vi "子界面-评定报告生成.vi"(0 "产品序号":string, 1 "测试人":string, 2 "部位":string, 3 "总面积":i32) -> (7 "写入数据库路径":path)   [LabVIEW 2018]
uses:
  <vilib>/Utility/NIReport.llb/Report Type.ctl
  <vilib>/addons/database/Connection.llb/DB Tools Open Connec (String).vi
  <vilib>/Utility/NIReport.llb/Append Report Text (str wrap).vi
  <vilib>/Utility/NIReport.llb/Append Report Text (num wrap).vi
  <vilib>/addons/database/_DB Variant To Data/Database Variant To Data.xnode
  <vilib>/Utility/NIReport.llb/NI_report.lvclass
  <vilib>/addons/database/NI_Database_API.lvlib
  <vilib>/Utility/NIReport.llb/NI_ReportGenerationCore.lvlib
panel:
  out "报告生成路径":path
  out "最大Z值":cluster{dbl}
  out "评定等级":string
  out "data":T1
  out "评定等级2":string caption="评定等级"
  out "缺陷占比(%)":dbl
  out "数值":dbl
  in  "返回 2":bool
  out "data 2":T1
  # "评定和分级结果"
  # "分层类"
  # "弥散类"
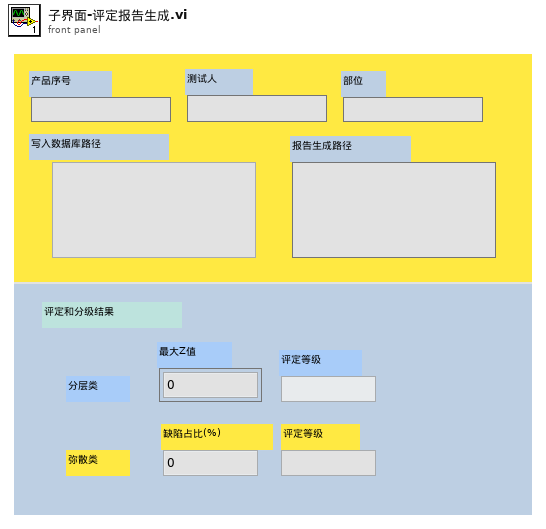
[diagram p1: front panel]
types:
  T1 = typedef "Z值ctl.ctl" = cluster{dbl}[]
  T2 = cluster{"position (Excel)":cluster{"row":i32, "column":i32}, "name (Excel)":string, "bookmark (Word)":string}
  T3 = typedef "NI_ReportGenerationCore.lvlib/Report Type.ctl" = enum16{"HTML", "Word", "Excel"}
  T4 = typedef "NI_Database_API.lvlib/Conn ObjectReference.ctl" = refnum<k1>
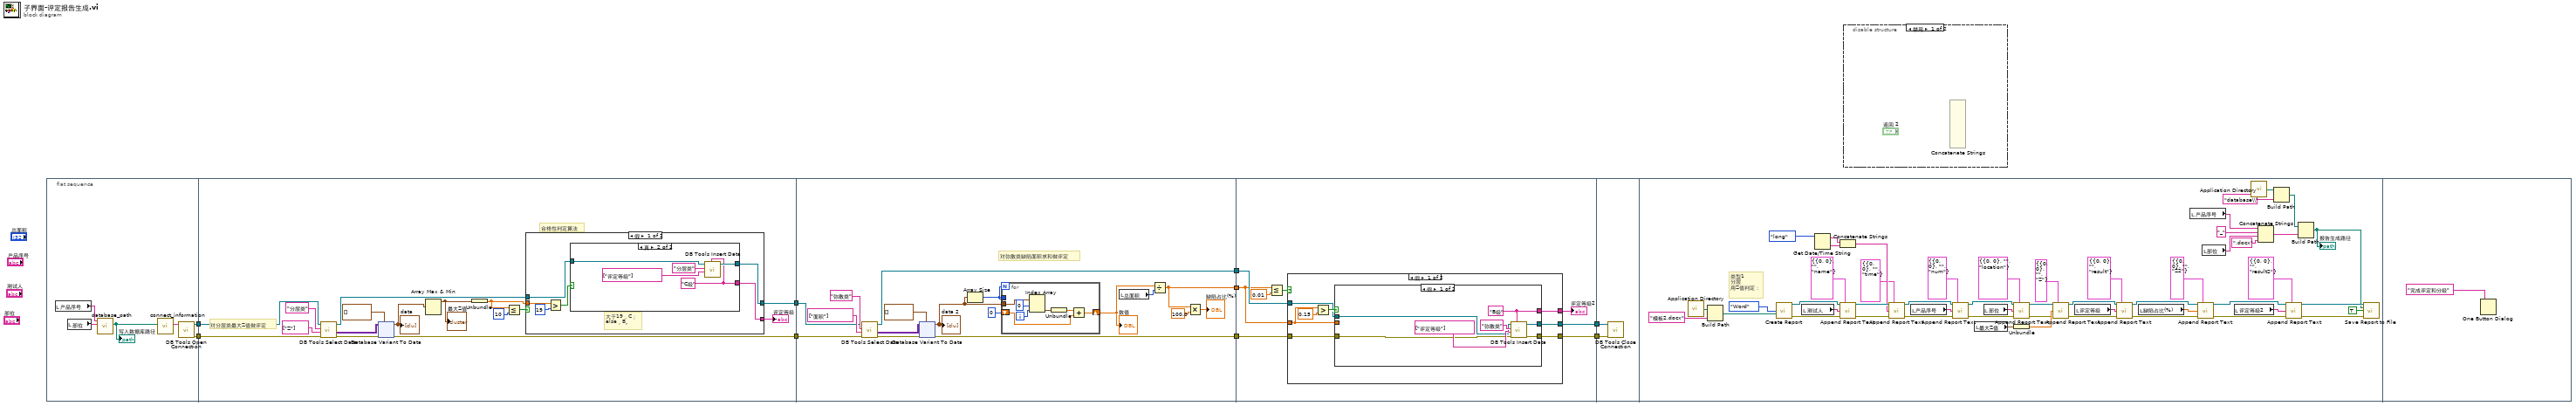
[diagram p0: block diagram]
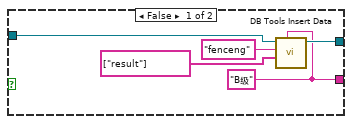
[diagram p2: hidden frame]
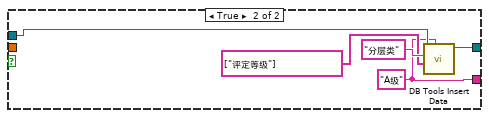
[diagram p3: hidden frame]
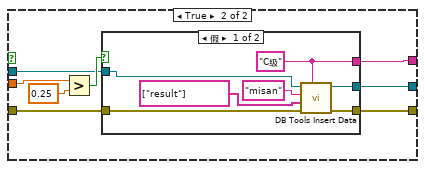
[diagram p4: hidden frame]
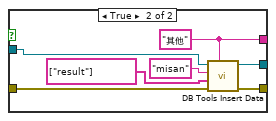
[diagram p5: hidden frame]
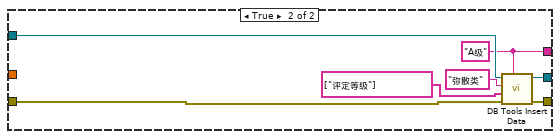
[diagram p6: hidden frame]
diagram:
  n1 = flat-sequence {
    tunnel: [w11] -> w9
    tunnel: [w10] -> w8
    tunnel: w9 -> [w25]
    tunnel: w8 -> [w28]
    tunnel: [w19] -> w7
    tunnel: [w17] -> w6
    tunnel: [w104] -> w5
    tunnel: w7 -> [w108]
    tunnel: w6 -> [w105]
    tunnel: [w103] -> w4
    tunnel: [w96] -> w3
    tunnel: w5 -> [w162]
    tunnel: w4 -> [w164]
    tunnel: [w163] -> w2
    tunnel: [w161] -> w1
    tunnel: w3 -> [w160]
    tunnel: w2 -> [w212]
    tunnel: w1 -> [w211]
    frame #0 {
      n2 = local read "产品序号"() -> (w13:string)
      n3 = local read "部位"() -> (w12:string)
      n4 = call "database_path.vi"("部位"=w12, "产品序号"=w13) -> ("database path"=w14:path)  [unwired: 9 in]
      "写入数据库路径" <- w14
      n5 = call "connect_information.vi"("路径"=w14) -> ("connect info"=w15:string)  [unwired: 10 in]
      n6 = call-poly <vilib>:"DB Tools Open Connection.vi"("connection information"=w15) -> ("error out"=w10:errorcluster, "connection reference"=w11:T4)  [unwired: 7 in]
    }
    frame #1 {
      # "合格性判定算法"
      # "对分层类最大Z值做评定"
      n7 = call <vilib>:"DB Tools Select Data.vi"("error in (no error)"=w28, "columns"=string[] ["Z"], "table"="分层类", "connection reference"=w25) -> ("error out"=w29:errorcluster, "data"=w27:variant[][], "connection reference out"=w20:T4)  [unwired: 2 in]
      n8 = xnode "Database Variant To Data"("database variant"=w27, "error in (no error)"=w29, "type"=T1 []) -> ("data"=w24:T1, "error out"=w17:errorcluster)
      "data" <- w24
      n9 = Array Max & Min(array=w24) -> (max value=w21:cluster{dbl})  [unwired: 3 out]
      "最大Z值" <- w21
      n10 = Unbundle(w21) -> (w18:dbl)
      n11 = Less Or Equal?(x=w18, y=10) -> (x <= y?=w22:bool)
      n12 = case shown="假" w22 {
        tunnel: w20 -> [w35 w52]
        tunnel: [w34 w49] -> w19
        tunnel: w18 -> [w33 _]
        tunnel: [w32 w48] -> w16
        frame False {
          # "大于19，C；\nelse，B。"
          n13 = Greater?(x=w33, y=19) -> (0:w36:bool)
          n14 = case shown="真" w36 {
            tunnel: w35 -> [w40 w44]
            tunnel: [w39 w45] -> w34
            tunnel: [w38 w43] -> w32
            frame False {
              w38 = "B级"
              n15 = call <vilib>:"DB Tools Insert Data.vi"("data"=w38, "columns"=string[] ["result"], "table"="fenceng", "connection reference"=w40) -> ("connection reference out"=w39:T4)  [unwired: 6 in, 1 out]
            }
            frame True {
              w43 = "C级"
              n16 = call <vilib>:"DB Tools Insert Data.vi"("data"=w43, "columns"=string[] ["评定等级"], "table"="分层类", "connection reference"=w44) -> ("connection reference out"=w45:T4)  [unwired: 6 in, 1 out]
            }
          }
        }
        frame True {
          w48 = "A级"
          n17 = call <vilib>:"DB Tools Insert Data.vi"("data"=w48, "columns"=string[] ["评定等级"], "table"="分层类", "connection reference"=w52) -> ("connection reference out"=w49:T4)  [unwired: 6 in, 1 out]
        }
      }
      "评定等级" <- w16
    }
    frame #2 {
      # "对弥散类缺陷面积求和做评定"
      n18 = call <vilib>:"DB Tools Select Data.vi"("error in (no error)"=w105, "columns"=string[] ["面积"], "table"="弥散类", "connection reference"=w108) -> ("error out"=w106:errorcluster, "data"=w107:variant[][], "connection reference out"=w103:T4)  [unwired: 2 in]
      n19 = xnode "Database Variant To Data"("database variant"=w107, "error in (no error)"=w106, "type"=T1 []) -> ("data"=w101:T1, "error out"=w104:errorcluster)
      "data 2" <- w101
      n20 = Array Size(array=w101) -> (size(s)=w100:i32)
      n21 = for {
        N: w100 -> [_]
        tunnel: w101 -> [w117]
        tunnel: w100 -> [_]
        shift-right: [w112] -> w98
        shift-left: 0 -> [w111]
        i -> [w115]
        n22 = Index Array(array=w117, index #1=0 ("索引 (列)"), index #2=w115) -> (element #2=w114:cluster{dbl})  [unwired: 1 out]
        n23 = Unbundle(w114) -> (w113:dbl)
        n24 = Add(x=w113, y=w111) -> (x+y=w112:dbl)
      }
      "数值" <- w98
      n25 = local read "总面积"() -> (w97:i32)
      n26 = Divide(x=w98, y=w97) -> (x/y=w96:dbl)
      n27 = Multiply(x=w96, y=100.0) -> (x*y=→"缺陷占比(%)":dbl)
    }
    frame #3 {
      n28 = Less Or Equal?(x=w160, y=0.01) -> (x <= y?=w166:bool)
      n29 = case shown="假" w166 {
        tunnel: w164 -> [w171 w208]
        tunnel: [w170 w207] -> w163
        tunnel: w162 -> [w168 w206]
        tunnel: [w169 w205] -> w161
        tunnel: w160 -> [w172 _]
        tunnel: [w167 w204] -> w159
        frame False {
          n30 = Greater?(x=w172, y=0.15) -> (0:w173:bool)
          n31 = case shown="假" w173 {
            tunnel: w172 -> [_ w187]
            tunnel: w171 -> [w179 w186]
            tunnel: [w178 w185] -> w170
            tunnel: [w177 w184] -> w169
            tunnel: w168 -> [w176 w183]
            tunnel: [w175 w182] -> w167
            frame False {
              w175 = "B级"
              n32 = call <vilib>:"DB Tools Insert Data.vi"("data"=w175, "error in (no error)"=w176, "columns"=string[] ["评定等级"], "table"="弥散类", "connection reference"=w179) -> ("error out"=w177:errorcluster, "connection reference out"=w178:T4)  [unwired: 5 in]
            }
            frame True {
              n33 = Greater?(x=w187, y=0.25) -> (0:w188:bool)
              n34 = case shown="假" w188 {
                tunnel: w186 -> [w194 w201]
                tunnel: [w193 w200] -> w185
                tunnel: [w192 w199] -> w184
                tunnel: w183 -> [w191 w198]
                tunnel: [w190 w197] -> w182
                frame False {
                  w190 = "C级"
                  n35 = call <vilib>:"DB Tools Insert Data.vi"("data"=w190, "error in (no error)"=w191, "columns"=string[] ["result"], "table"="misan", "connection reference"=w194) -> ("error out"=w192:errorcluster, "connection reference out"=w193:T4)  [unwired: 5 in]
                }
                frame True {
                  w197 = "其他"
                  n36 = call <vilib>:"DB Tools Insert Data.vi"("data"=w197, "error in (no error)"=w198, "columns"=string[] ["result"], "table"="misan", "connection reference"=w201) -> ("error out"=w199:errorcluster, "connection reference out"=w200:T4)  [unwired: 5 in]
                }
              }
            }
          }
        }
        frame True {
          w204 = "A级"
          n37 = call <vilib>:"DB Tools Insert Data.vi"("data"=w204, "error in (no error)"=w206, "columns"=string[] ["评定等级"], "table"="弥散类", "connection reference"=w208) -> ("error out"=w205:errorcluster, "connection reference out"=w207:T4)  [unwired: 5 in]
        }
      }
      "评定等级2" <- w159
    }
    frame #4 {
      n38 = call <vilib>:"DB Tools Close Connection.vi"("error in (no error)"=w211, "connection reference"=w212) -> ()  [unwired: 5 in, 1 out]
    }
    frame #5 {
      # "类型1\n分层\n用Z值判定："
      n39 = call <vilib>:"Application Directory.vi"() -> ("Application Directory"=w264:path)
      n40 = Build Path(base path=w264, name or relative path="模板2.docx") -> (appended path=w263:path)
      n41 = call <vilib>:"Create Report.vi"("report type"=Report_Type."Word" ("Report Type"), "template (empty)"=w263) -> ("report out"=w246:refnum<class "NI_report.lvclass">, "error out"=w245:errorcluster)  [unwired: 12 in]
      n42 = local read "测试人"() -> (w244:string)
      n43 = Get Date/Time String(date format (0)=enum16{"short", "long", "abbreviated"}."long" ("日期格式(0)")) -> (date string=w252:string, time string=w254:string)  [unwired: 2 in]
      n44 = Concatenate Strings(w252, w254) -> (w253:string)
      n45 = call-poly <vilib>:"Append Report Text.vi"("report in"=w246, "MS Office parameters"=T2 {"position (Excel)"={"row"=0, "column"=0}, "name (Excel)"="", "bookmark (Word)"="name"}, "text"=w244, "error in (no error)"=w245) -> ("report out"=w257:refnum<class "NI_report.lvclass">, "error out"=w258:errorcluster)  [unwired: 8 in, 2 out]
      n46 = call-poly <vilib>:"Append Report Text.vi"("report in"=w257, "MS Office parameters"=T2 {"position (Excel)"={"row"=0, "column"=0}, "name (Excel)"="", "bookmark (Word)"="time"}, "text"=w253, "error in (no error)"=w258) -> ("report out"=w255:refnum<class "NI_report.lvclass">, "error out"=w256:errorcluster)  [unwired: 8 in, 2 out]
      n47 = local read "产品序号"() -> (w243:string)
      n48 = call-poly <vilib>:"Append Report Text.vi"("report in"=w255, "MS Office parameters"=T2 {"position (Excel)"={"row"=0, "column"=0}, "name (Excel)"="", "bookmark (Word)"="num"}, "text"=w243, "error in (no error)"=w256) -> ("report out"=w259:refnum<class "NI_report.lvclass">, "error out"=w260:errorcluster)  [unwired: 8 in, 2 out]
      n49 = local read "最大Z值"() -> (w236:cluster{dbl})
      n50 = local read "部位"() -> (w242:string)
      n51 = call-poly <vilib>:"Append Report Text.vi"("report in"=w259, "MS Office parameters"=T2 {"position (Excel)"={"row"=0, "column"=0}, "name (Excel)"="", "bookmark (Word)"="location"}, "text"=w242, "error in (no error)"=w260) -> ("report out"=w232:refnum<class "NI_report.lvclass">, "error out"=w231:errorcluster)  [unwired: 8 in, 2 out]
      n52 = Unbundle(w236) -> (w237:dbl)
      n53 = call-poly <vilib>:"Append Report Text.vi"("report in"=w232, "MS Office parameters"=T2 {"position (Excel)"={"row"=0, "column"=0}, "name (Excel)"="", "bookmark (Word)"="Z"}, "text"=w237, "error in (no error)"=w231) -> ("report out"=w230:refnum<class "NI_report.lvclass">, "error out"=w229:errorcluster)  [unwired: 8 in, 2 out]
      n54 = local read "评定等级"() -> (w235:string)
      n55 = call-poly <vilib>:"Append Report Text.vi"("report in"=w230, "MS Office parameters"=T2 {"position (Excel)"={"row"=0, "column"=0}, "name (Excel)"="", "bookmark (Word)"="result"}, "text"=w235, "error in (no error)"=w229) -> ("report out"=w228:refnum<class "NI_report.lvclass">, "error out"=w227:errorcluster)  [unwired: 8 in, 2 out]
      n56 = local read "缺陷占比(%)"() -> (w234:dbl)
      n57 = local read "产品序号"() -> (w220:string)
      n58 = call-poly <vilib>:"Append Report Text.vi"("report in"=w228, "MS Office parameters"=T2 {"position (Excel)"={"row"=0, "column"=0}, "name (Excel)"="", "bookmark (Word)"="Z2"}, "text"=w234, "error in (no error)"=w227) -> ("report out"=w226:refnum<class "NI_report.lvclass">, "error out"=w225:errorcluster)  [unwired: 8 in, 2 out]
      n59 = local read "部位"() -> (w219:string)
      n60 = local read "评定等级2"() -> (w233:string)
      n61 = call <vilib>:"Application Directory.vi"() -> ("Application Directory"=w215:path)
      n62 = Concatenate Strings(w220, "_" ("名称或相对路径"), w219, ".docx" ("名称或相对路径")) -> (w223:string)
      n63 = Build Path(base path=w215, name or relative path="database\\" ("名称或相对路径")) -> (appended path=w213:path)
      n64 = call-poly <vilib>:"Append Report Text.vi"("report in"=w226, "MS Office parameters"=T2 {"position (Excel)"={"row"=0, "column"=0}, "name (Excel)"="", "bookmark (Word)"="result2"}, "text"=w233, "error in (no error)"=w225) -> ("report out"=w218:refnum<class "NI_report.lvclass">, "error out"=w217:errorcluster)  [unwired: 8 in, 2 out]
      n65 = Build Path(base path=w213, name or relative path=w223) -> (appended path=w216:path)
      "报告生成路径" <- w216
      n66 = call-dynamic "Save Report to File.vi"("report in"=w218, "report file path"=w216, "prompt to replace? (F)"=TRUE, "error in (no error)"=w217) -> ()  [unwired: 10 in, 2 out]
    }
    frame #6 {
      n67 = One Button Dialog(message="完成评定和分级" ("消息")) -> ()  [unwired: 1 in, 1 out]
    }
  }
  n68 = disable-structure shown="禁用" {
    frame Disabled {
      n69 = Concatenate Strings() -> ()  [unwired: 12 in, 1 out]
    }
    frame Enabled {
    }
  }
